vi "percentage.vi"(11 "Numeric":sgl) -> (1 "Boolean 2":bool, 2 "Boolean 3":bool, 3 "Boolean 4":bool, 4 "Boolean":bool)   [LabVIEW 2015]
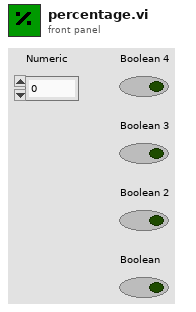
[diagram p1: front panel]
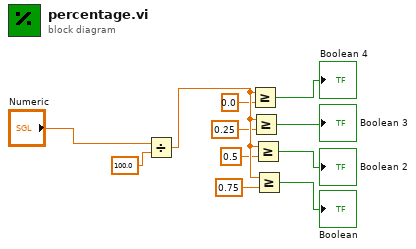
[diagram p0: block diagram]
diagram:
  n1 = Divide(x="Numeric", y=sgl 100.0) -> (x/y=w6:sgl)
  n2 = Greater Or Equal?(x=w6, y=0.0) -> (x >= y?=→"Boolean 4":bool)
  n3 = Greater Or Equal?(x=w6, y=0.25) -> (x >= y?=→"Boolean 3":bool)
  n4 = Greater Or Equal?(x=w6, y=0.5) -> (x >= y?=→"Boolean 2":bool)
  n5 = Greater Or Equal?(x=w6, y=0.75) -> (x >= y?=→"Boolean":bool)
